vi "设置UI.vi"() -> ()   [LabVIEW 2016, in "Alarm interface.lvlib" / "短信语音库.lvlib"]
uses:
  <vilib>/Utility/config.llb/NI_LVConfig.lvlib
panel:
  in  "PN3":T1
  in  "PN2":T1
  in  "PN1":T1
  in  "关闭":bool
  in  "启用":bool
  out "内容":string
  in  "测试":bool
  out "error out":errorcluster caption="错误输出"
  out "body":string caption="体部"
  out "headers":string caption="头部"
  in  "站点":string
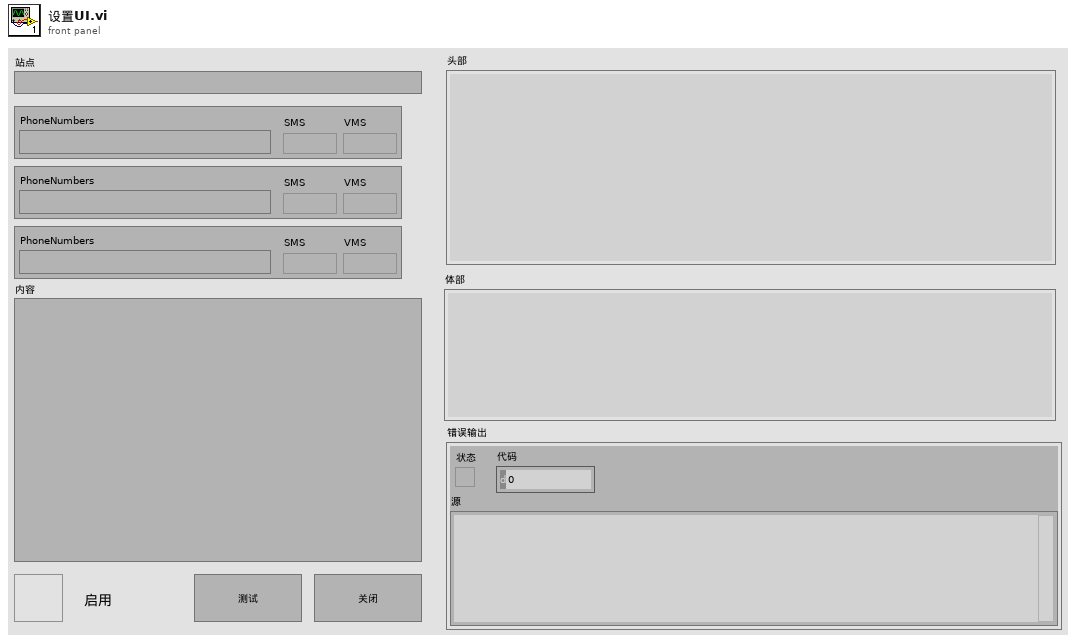
[diagram p1: front panel]
types:
  T1 = cluster{"PhoneNumbers":string, "SMS":bool, "VMS":bool}
  T2 = typedef "NI_LVConfig.lvlib/Config Data RefNum.ctl" = refnum<k1>
  T3 = enum32{"Invalid", "Standard", "Closed", "Hidden", "Minimized", "Maximized"}
  T4 = cluster{"PhoneNumbers":string, "SMS":bool, "VMS":bool}[]
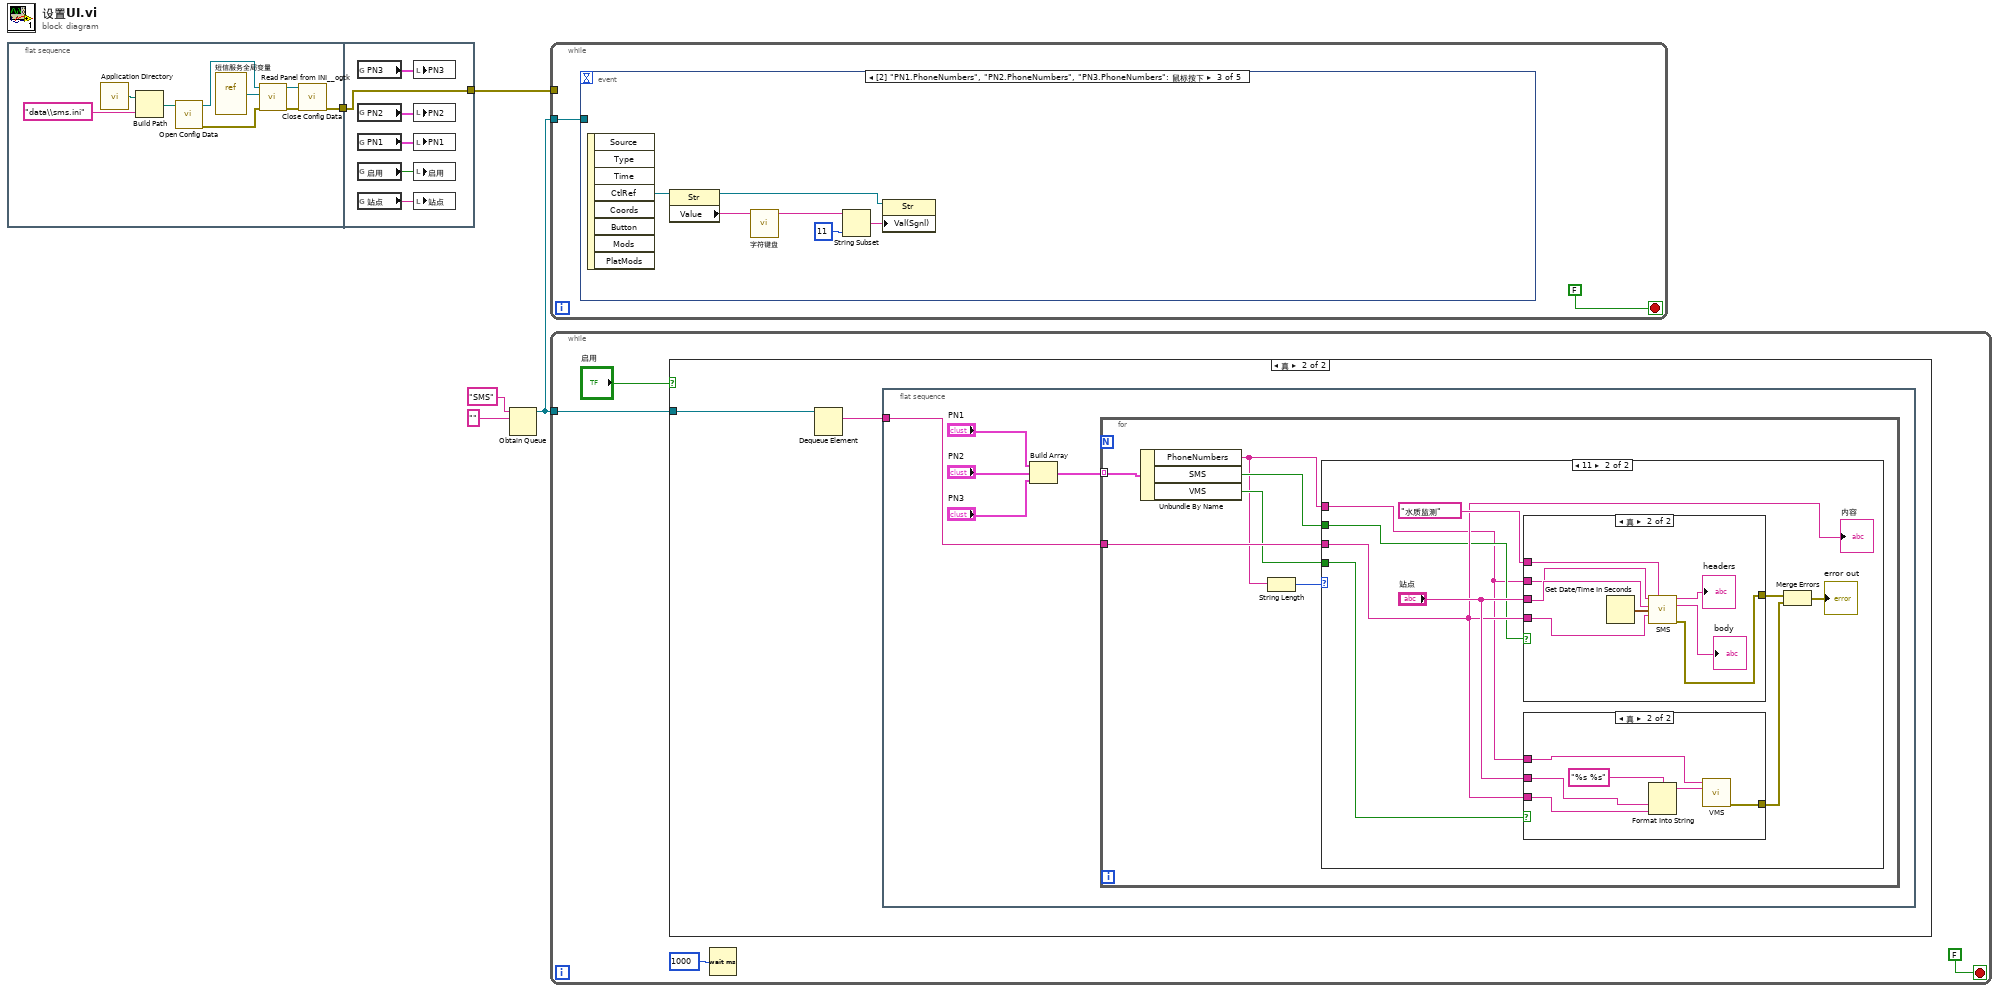
[diagram p0: block diagram]
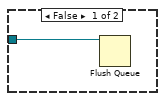
[diagram p2: hidden frame]
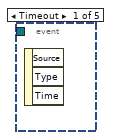
[diagram p6: hidden frame]
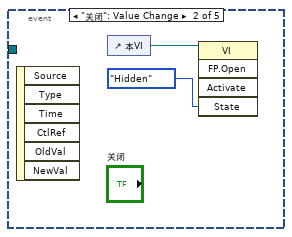
[diagram p7: hidden frame]
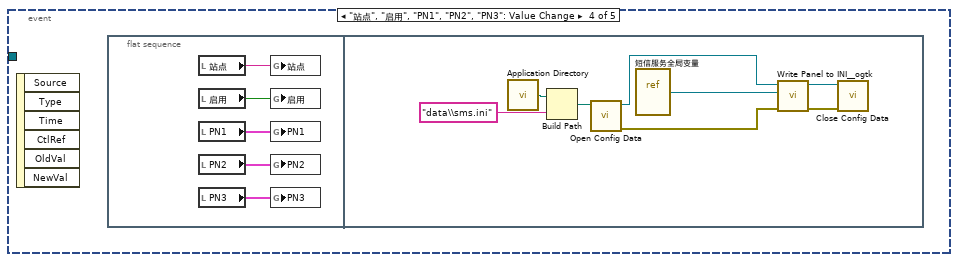
[diagram p8: hidden frame]
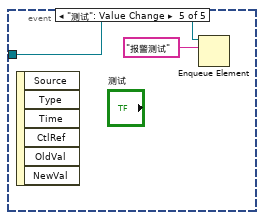
[diagram p9: hidden frame]
diagram:
  n1 = flat-sequence {
    tunnel: [w6] -> w4
    tunnel: [w20] -> w5
    tunnel: w4 -> [w20]
    frame #0 {
      n2 = call <vilib>:"Application Directory.vi"() -> ("Application Directory"=w12:path)
      n3 = Build Path(base path=w12, name or relative path="data\\sms.ini" ("名称或相对路径")) -> (appended path=w13:path)
      n4 = call <vilib>:"Open Config Data.vi"("configuration file path"=w13) -> ("error out"=w8:errorcluster, "refnum"=w7:T2)  [unwired: 8 in, 1 out]
      n5 = vi-ref "短信服务全局变量.vi"() -> (w11:refnum<vi>)
      n6 = call <userlib>:"Read Panel from INI__ogtk.vi"("error in (no error)"=w8, "VI ref"=w11, "refnum"=w7) -> ("error out"=w10:errorcluster, "refnum out"=w9:T2)  [unwired: 7 in]
      n7 = call <vilib>:"Close Config Data.vi"("error in (no error)"=w10, "refnum"=w9) -> ("error out"=w6:errorcluster)  [unwired: 8 in, 1 out]
    }
    frame #1 {
      n8 = global read "短信服务全局变量.vi" "PN3"() -> (w15:T1)
      n9 = global read "短信服务全局变量.vi" "PN2"() -> (w16:T1)
      n10 = global read "短信服务全局变量.vi" "PN1"() -> (w17:T1)
      n11 = global read "短信服务全局变量.vi" "启用"() -> (w18:bool)
      n12 = global read "短信服务全局变量.vi" "站点"() -> (w19:string)
      n13 = local write "PN3"(w15) -> ()
      n14 = local write "PN2"(w16) -> ()
      n15 = local write "PN1"(w17) -> ()
      n16 = local write "启用"(w18) -> ()
      n17 = local write "站点"(w19) -> ()
    }
  }
  n18 = Obtain Queue(name (unnamed)="SMS" ("名称（未命名）"), element data type="" ("名称（未命名）")) -> (queue out=w1:refnum<queue>)  [unwired: 3 in, 2 out]
  n19 = while {
    tunnel: w5 -> [_]
    tunnel: w1 -> [w21]
    stop <- FALSE stop-if-true
    n20 = event shown="[2] \"PN1.PhoneNumbers\", \"PN2.PhoneNumbers\", \"PN3.PhoneNumbers\": 鼠标按下" {
      selector: _ -> [_ _ _ _ _]
      dyn-events: _ -> [_ _ _ _ _]
      timeout: _ -> [_ _ _ _ _]
      tunnel: w21 -> [_ _ _ _ w45]
      event Timeout {
        n21 = event-data() -> ()  [unwired: 1 in, 3 out]
      }
      event "关闭": Value Change {
        n22 = event-data() -> ()  [unwired: 1 in, 6 out]
        n23 = control-ref of="本VI"() -> (w23:refnum<vi>)
        n24 = invoke class="VI" method="FP.Open"(reference=w23, "State"=T3."Hidden" ("状态")) -> ()  [unwired: 3 in, 5 out]
      }
      event "PN1.PhoneNumbers", "PN2.PhoneNumbers", "PN3.PhoneNumbers": Mouse Down {
        n25 = event-data() -> ("CtlRef"=w30:refnum<vi>)  [unwired: 1 in, 7 out]
        n26 = property class="Str"(reference=w30) -> (reference out=w27:refnum<vi>, "Value"=w29:string)  [unwired: 1 in, 1 out]
        n27 = call "字符键盘.vi"("Old String"=w29) -> ("String"=w28:string)  [unwired: 10 in]
        n28 = String Subset(string=w28, length (rest)=11 ("长度（剩余）")) -> (substring=w26:string)  [unwired: 1 in]
        n29 = property class="Str"(reference=w27, "Val(Sgnl)"=w26) -> ()  [unwired: 1 in, 2 out]
      }
      event "站点", "启用", "PN1", "PN2", "PN3": Value Change {
        n30 = event-data() -> ()  [unwired: 1 in, 6 out]
        n31 = flat-sequence {
          frame #0 {
            n32 = local read "站点"() -> (w35:string)
            n33 = local read "启用"() -> (w33:bool)
            n34 = local read "PN1"() -> (w34:T1)
            n35 = local read "PN2"() -> (w32:T1)
            n36 = local read "PN3"() -> (w31:T1)
            n37 = global write "短信服务全局变量.vi" "站点"(w35) -> ()
            n38 = global write "短信服务全局变量.vi" "启用"(w33) -> ()
            n39 = global write "短信服务全局变量.vi" "PN1"(w34) -> ()
            n40 = global write "短信服务全局变量.vi" "PN2"(w32) -> ()
            n41 = global write "短信服务全局变量.vi" "PN3"(w31) -> ()
          }
          frame #1 {
            n42 = call <vilib>:"Application Directory.vi"() -> ("Application Directory"=w38:path)
            n43 = Build Path(base path=w38, name or relative path="data\\sms.ini" ("名称或相对路径")) -> (appended path=w37:path)
            n44 = call <vilib>:"Open Config Data.vi"("configuration file path"=w37) -> ("error out"=w42:errorcluster, "refnum"=w43:T2)  [unwired: 8 in, 1 out]
            n45 = vi-ref "短信服务全局变量.vi"() -> (w39:refnum<vi>)
            n46 = call <userlib>:"Write Panel to INI__ogtk.vi"("error in (no error)"=w42, "VI ref"=w39, "refnum"=w43) -> ("error out"=w40:errorcluster, "refnum out"=w41:T2)  [unwired: 7 in]
            n47 = call <vilib>:"Close Config Data.vi"("error in (no error)"=w40, "refnum"=w41) -> ()  [unwired: 8 in, 2 out]
          }
        }
      }
      event "测试": Value Change {
        n48 = event-data() -> ()  [unwired: 1 in, 6 out]
        n49 = Enqueue Element(queue=w45, element="报警测试" ("内容")) -> ()  [unwired: 2 in, 3 out]
      }
    }
  }
  n50 = while {
    tunnel: w1 -> [w47]
    stop <- FALSE stop-if-true
    n51 = case shown="真" "启用" {
      tunnel: w47 -> [w50 w52]
      frame False {
        n52 = Flush Queue(queue=w50) -> ()  [unwired: 1 in, 3 out]
      }
      frame True {
        n53 = Dequeue Element(queue=w52) -> (element=w51:string)  [unwired: 2 in, 3 out]
        n54 = flat-sequence {
          tunnel: w51 -> [w57]
          frame #0 {
            n55 = Build Array("PN1", "PN2", "PN3") -> (w53:T4)
            n56 = for {
              tunnel: w57 -> [w63]
              tunnel: w53 -> [w62] mode=indexing
              n57 = Unbundle By Name(w62) -> ("PhoneNumbers"=w59:string, "SMS"=w61:bool, "VMS"=w60:bool)
              n58 = String Length(string=w59) -> (length=w58:i32)
              n59 = case shown="11" w58 {
                tunnel: w63 -> [_ w67]
                tunnel: w61 -> [_ w66]
                tunnel: w60 -> [_ w65]
                tunnel: w59 -> [_ w64]
                frame 0, Default {
                }
                frame 11 {
                  n60 = case shown="真" w66 {
                    tunnel: "水质监测" ("SignName") -> [_ w86]
                    tunnel: [_ w82] -> w71
                    tunnel: "站点" -> [_ w81]
                    tunnel: w67 -> [_ w80]
                    tunnel: w64 -> [_ w79]
                    frame False {
                    }
                    frame True {
                      n61 = Get Date/Time In Seconds() -> (seconds since 1Jan1904=w85:timestamp)
                      n62 = call "SMS.vi"("PhoneNumbers"=w79, "SignName"=w86, "站点"=w81, "时间标识"=w85, "内容"=w80) -> ("headers"=→"headers":string, "body"=→"body":string, "error out"=w82:errorcluster)  [unwired: 8 in]
                    }
                  }
                  n63 = case shown="真" w65 {
                    tunnel: [_ w78] -> w69
                    tunnel: "站点" -> [_ w76]
                    tunnel: w67 -> [_ w75]
                    tunnel: w64 -> [_ w73]
                    frame False {
                    }
                    frame True {
                      n64 = Format Into String(format string="%s %s" ("格式字符串"), w76, w75) -> (resulting string=w74:string)  [unwired: 2 in, 1 out]
                      n65 = call "VMS.vi"("PhoneNumbers"=w73, "内容"=w74) -> ("error out"=w78:errorcluster)  [unwired: 11 in, 2 out]
                    }
                  }
                  n66 = Merge Errors(w71, w69) -> (→"error out":errorcluster)
                  "内容" <- w67
                }
              }
            }
          }
        }
      }
    }
    n67 = Wait (ms)(milliseconds to wait=u32 1000 ("等待时间（毫秒）")) -> ()  [unwired: 1 out]
  }
